vi "Handle GroupData.vi"(7 "Source ID":u32, 8 "GroupData":T1, 9 "Sequence":u32, 10 "ChannelService":refnum<class "ChannelService.lvclass">, 11 "Subscription Loop Data in":T2) -> (0 "error out":errorcluster, 3 "Subscription Loop Data":T2)   [LabVIEW 2020, in "Vecto.lvlib" / "RemoteDataService.lvclass"]
uses:
  RemoteDataService.lvclass
  Subscription Loop Data.ctl
  Subscription Group Info.ctl
  Group/Group.lvclass
  SubscribedDataHandler/SubscribedDataHandler.lvclass
  proto/GroupData/Data.ctl
  ChannelService/ChannelService.lvclass
  Group DBL/Group DBL.lvclass
  C:/dev/lv20CE/relink/lv-vecto/Vecto/Group/Group.lvclass
  <vilib>/Utility/miscctls.llb/LVMapReplaceAction.ctl
  Vecto.lvlib
  proto/GroupData/GroupData.lvlib
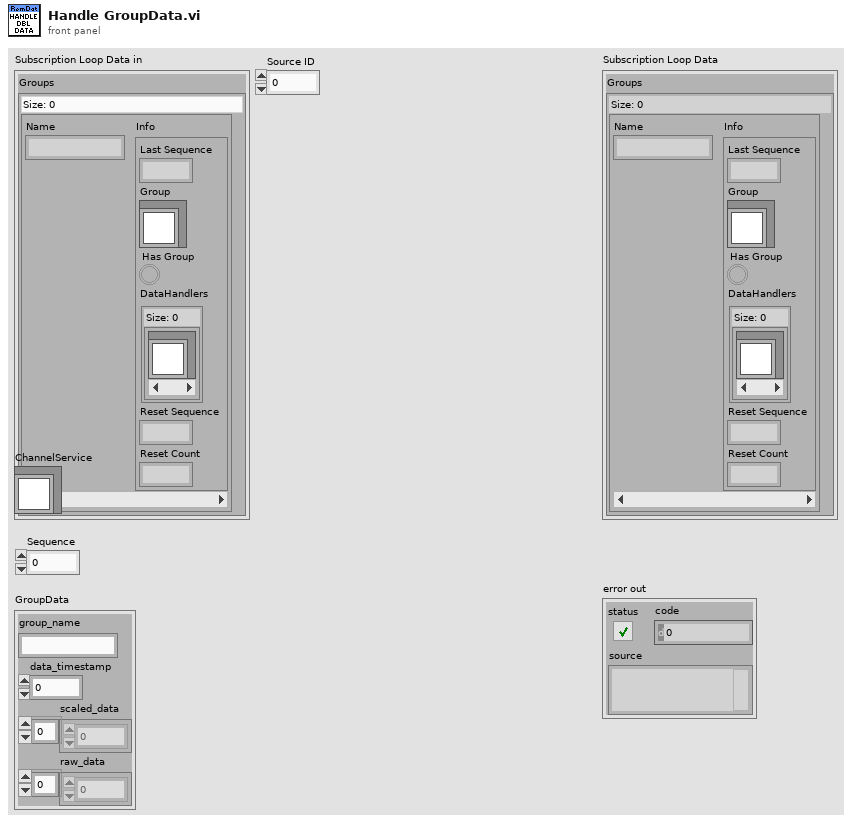
[diagram p1: front panel]
types:
  T1 = typedef "GroupData.lvlib/Data.ctl" = cluster{"group_name":string, "data_timestamp":i64, "scaled_data":dbl[], "raw_data":dbl[]}
  T2 = typedef "Vecto.lvlib/RemoteDataService.lvclass/Subscription Loop Data.ctl" = cluster{"Groups":map{string, T3}}
  T3 = typedef "Vecto.lvlib/RemoteDataService.lvclass/Subscription Group Info.ctl" = cluster{"Last Sequence":u32, "Group":refnum<class "Group.lvclass">, "Has Group":bool, "DataHandlers":set{refnum<class "SubscribedDataHandler.lvclass">}, "Reset Sequence":u32, "Reset Count":u32}
  T4 = typedef "LVMapReplaceAction.ctl" = enum32{"Modify Entry only if found", "Add or Modify Entry", "Delete Entry"}
  T5 = set{refnum<class "SubscribedDataHandler.lvclass">}
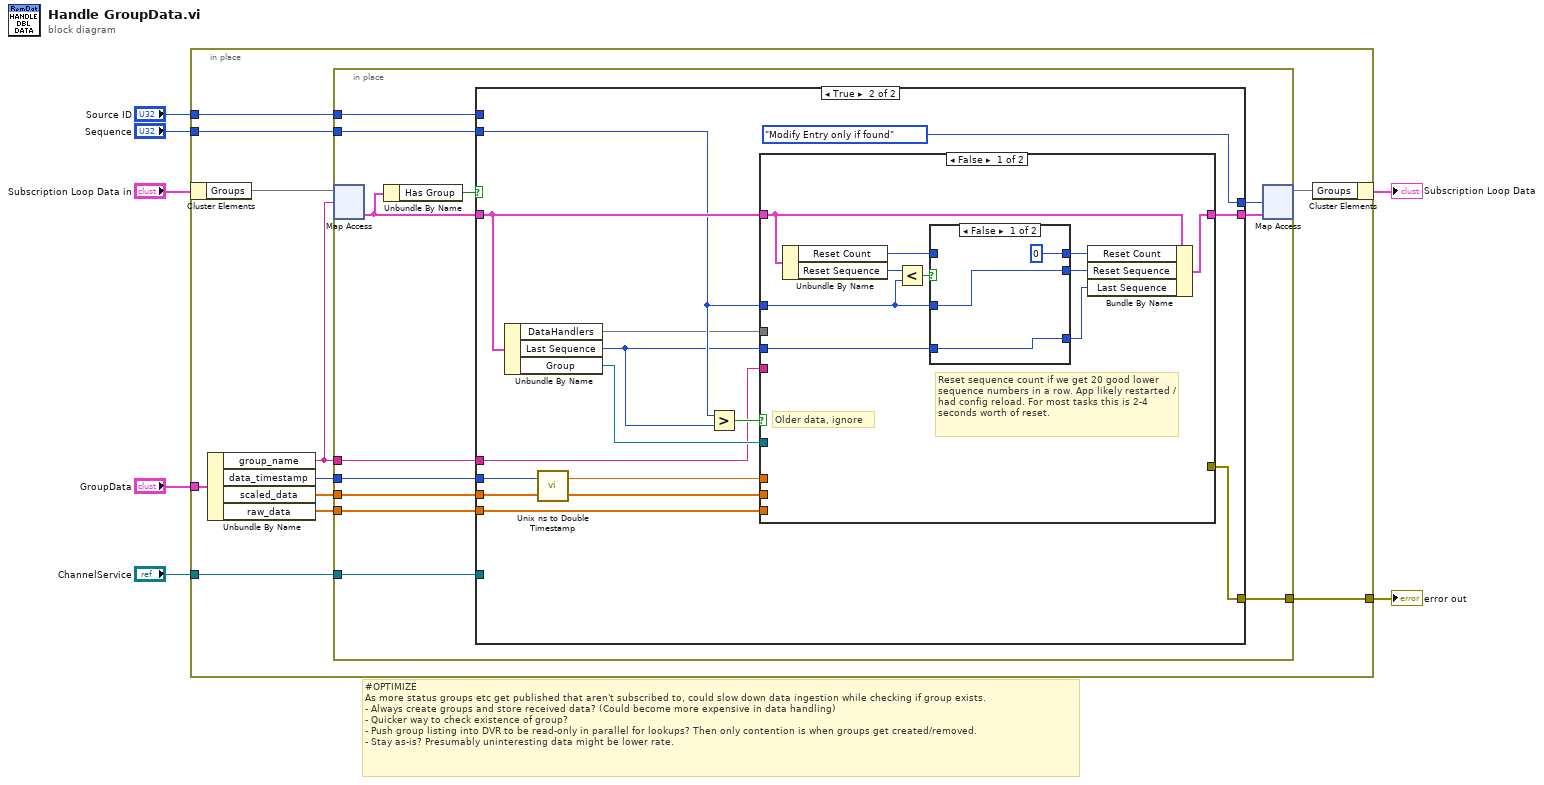
[diagram p0: block diagram]
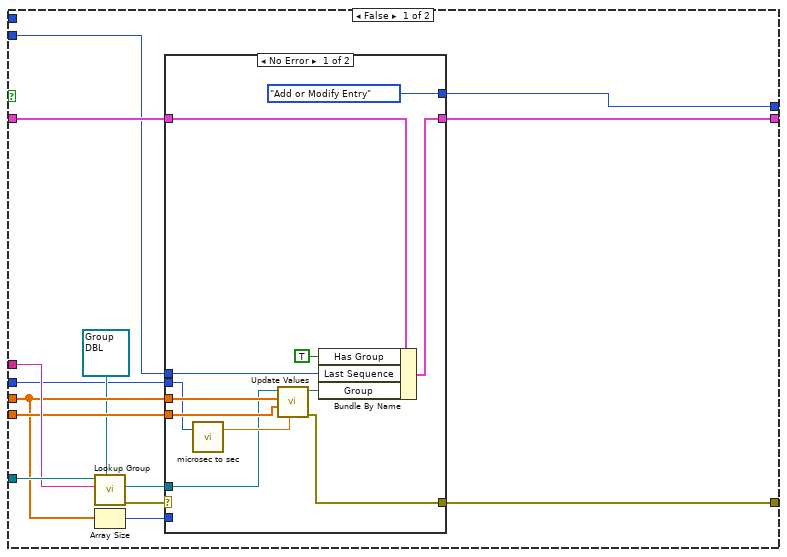
[diagram p2: hidden frame]
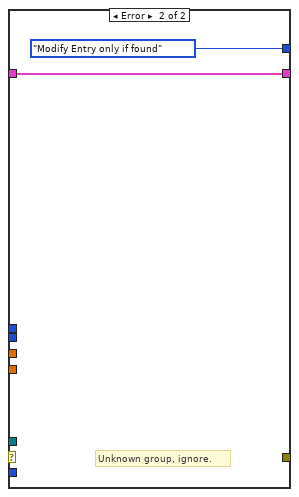
[diagram p3: hidden frame]
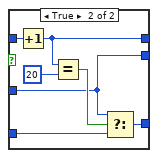
[diagram p4: hidden frame]
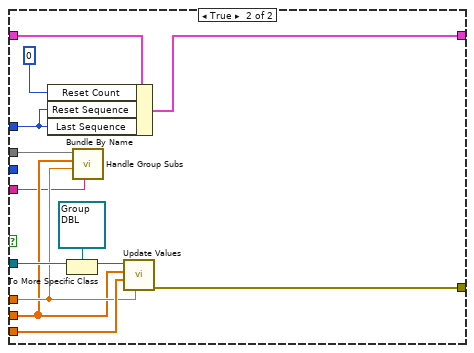
[diagram p5: hidden frame]
diagram:
  # "#OPTIMIZE\nAs more status groups etc get published that aren't subscribed to, could slow down data ingestion while checking if group exists.\n- Always create groups and store received data? (Could become more expensive in data handling)\n- Quicker way to check existence of group?\n- Push group listing into DVR to be read-only in parallel for lookups? Then only contention is when groups get created/removed.\n- Stay as-is? Presumably uninteresting data might be lower rate."
  n1 = in-place {
    in-place-border: "GroupData" -> [w8]
    in-place-border: "ChannelService" -> [w17]
    in-place-border: "Sequence" -> [w12]
    in-place-border: "Source ID" -> [w11]
    in-place-border: [w9] -> w2
    n2 = in-place-cluster #1("Subscription Loop Data in") -> ("Groups"=w18:map{string, T3})
    n3 = Unbundle By Name(w8) -> ("group_name"=w16:string, "data_timestamp"=w13:i64, "scaled_data"=w14:dbl[], "raw_data"=w15:dbl[])
    n4 = in-place {
      in-place-border: w17 -> [w30]
      in-place-border: w16 -> [w29]
      in-place-border: w15 -> [w28]
      in-place-border: w14 -> [w27]
      in-place-border: w13 -> [w26]
      in-place-border: w12 -> [w25]
      in-place-border: w11 -> [w24]
      in-place-border: [w22] -> w9
      n5 = in-place-map #2(w18, w16) -> (w20:T3)  [unwired: 1 in, 1 out]
      n6 = Unbundle By Name(w20) -> ("Has Group"=w19:bool)
      n7 = case shown="True" w19 {
        tunnel: w20 -> [w39 w67]
        tunnel: w30 -> [w44 _]
        tunnel: w29 -> [w42 w61]
        tunnel: w28 -> [w37 w68]
        tunnel: w27 -> [w36 w69]
        tunnel: w26 -> [w31 w70]
        tunnel: w25 -> [w38 w65]
        tunnel: w24 -> [_ _]
        tunnel: [w35 w66] -> w23
        tunnel: [w34 w64] -> w22
        tunnel: [w33 LVMapReplaceAction."Modify Entry only if found" ("action")] -> w21
        frame False {
          n8 = call "Lookup Group.vi"("Group Type (Abstract)"=refnum<class "Group DBL.lvclass"> refnum ("Vecto.lvlib:Group.lvclass"), "Group Name"=w42, "ChannelService in"=w44) -> ("error out"=w43:errorcluster, "Group"=w41:refnum<class "Group DBL.lvclass">)  [unwired: 6 in, 1 out]
          n9 = Array Size(array=w36) -> (size(s)=w40:i32)
          n10 = case shown="No Error" w43 {
            tunnel: w41 -> [w47 _]
            tunnel: w40 -> [_ _]
            tunnel: w39 -> [w46 w57]
            tunnel: w38 -> [w56 _]
            tunnel: w37 -> [w55 _]
            tunnel: w36 -> [w54 _]
            tunnel: [w53 w57] -> w35
            tunnel: [w52 _] -> w34
            tunnel: [LVMapReplaceAction."Add or Modify Entry" ("action") LVMapReplaceAction."Modify Entry only if found" ("action")] -> w33
            tunnel: w31 -> [w49 _]
            frame No Error {
              n11 = call "microsec to sec.vi"("data_timestamp us"=w49) -> ("timestamp s"=w48:dbl)  [unwired: 2 in]
              n12 = call "Update Values.vi"("Timestamp (Now)"=w48, "Raw Values (N/A)"=w55, "Values"=w54, "Group in"=w47) -> ("error out"=w52:errorcluster, "Group out"=w51:refnum<class "Group DBL.lvclass">)  [unwired: 6 in]
              n13 = Bundle By Name(cluster=w46, "Has Group"=TRUE, "Last Sequence"=w56, "Group"=w51) -> (w53:T3)
            }
            frame Error {
              # "Unknown group, ignore."
            }
          }
        }
        frame True {
          n14 = Unbundle By Name(w67) -> ("DataHandlers"=w60:T5, "Last Sequence"=w59:u32, "Group"=w72:refnum<class "Group.lvclass">)
          n15 = call "Unix ns to Double Timestamp.vi"("unix ns"=w70) -> ("Timestamp"=w62:dbl)  [unwired: 2 in]
          n16 = Greater?(x=w65, y=w59) -> (0:w71:bool)
          n17 = case shown="False" w71 {
            tunnel: w72 -> [_ w105]
            tunnel: w62 -> [_ w98]
            tunnel: w69 -> [_ w97]
            tunnel: w68 -> [_ w104]
            tunnel: w67 -> [w78 w103]
            tunnel: [w76 w102] -> w66
            tunnel: w65 -> [w79 w94]
            tunnel: [_ w101] -> w64
            tunnel: w61 -> [_ w96]
            tunnel: w60 -> [_ w95]
            tunnel: w59 -> [w80 _]
            frame False {
              # "Reset sequence count if we get 20 good lower sequence numbers in a row. App likely restarted / had config reload. For most tasks this is 2-4 seconds worth of reset."
              # "Older data, ignore"
              n18 = Unbundle By Name(w78) -> ("Reset Count"=w81:u32, "Reset Sequence"=w74:u32)
              n19 = Less?(x=w74, y=w79) -> (x < y?=w82:bool)
              n20 = case shown="False" w82 {
                tunnel: w81 -> [_ w92]
                tunnel: w80 -> [w84 w90]
                tunnel: w79 -> [w83 w86]
                tunnel: [w84 w88] -> w75
                tunnel: [u32 0 w87] -> w77
                tunnel: [w83 w86] -> w73
                frame False {
                }
                frame True {
                  n21 = Increment(x=w92) -> (x+1=w87:u32)
                  n22 = Equal?(x=w87, y=u32 20) -> (x = y?=w89:bool)
                  n23 = Select(t=w86, s=w89, f=w90) -> (s? t:f=w88:u32)
                }
              }
              n24 = Bundle By Name(cluster=w78, "Reset Count"=w77, "Reset Sequence"=w73, "Last Sequence"=w75) -> (w76:T3)
            }
            frame True {
              n25 = Bundle By Name(cluster=w103, "Reset Count"=u32 0, "Reset Sequence"=w94, "Last Sequence"=w94) -> (w102:T3)
              n26 = To More Specific Class(target class=refnum<class "Group DBL.lvclass"> refnum ("Group in"), reference=w105) -> (specific class reference=w100:refnum<class "Group DBL.lvclass">)  [unwired: 1 in, 1 out]
              n27 = call "Handle Group Subs.vi"("Group"=w96, "Timestamp"=w98, "Data"=w97, "Data Handlers"=w95) -> ()  [unwired: 8 in]
              n28 = call "Update Values.vi"("Timestamp (Now)"=w98, "Raw Values (N/A)"=w104, "Values"=w97, "Group in"=w100) -> ("error out"=w101:errorcluster)  [unwired: 6 in, 1 out]
            }
          }
        }
      }
      n29 = in-place-map #2(w23, w21) -> (w10:map{string, T3})  [unwired: 2 out]
    }
    n30 = in-place-cluster #1("Groups"=w10) -> (→"Subscription Loop Data":T2)
  }
  "error out" <- w2
